vi "DAE Spring Pendulum Simulation_Func.vi"(2 "data":variant, 3 "t":dbl, 4 "X'":dbl[](array[numeric]), 5 "X":dbl[](array[numeric])) -> (0 "error out":errorcluster, 1 "F(X,X',t)":dbl[](array[numeric]))   [LabVIEW 2023]
doc: "DAE Spring Pendulum Simulation Function"
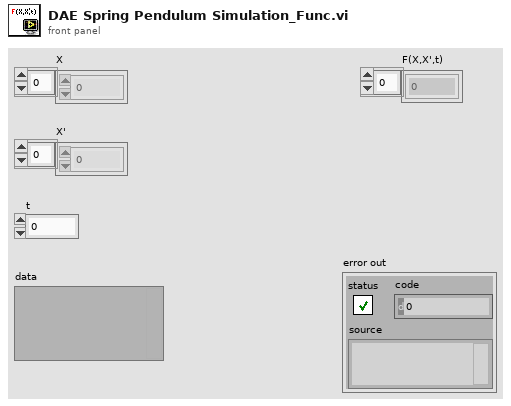
[diagram p1: front panel]
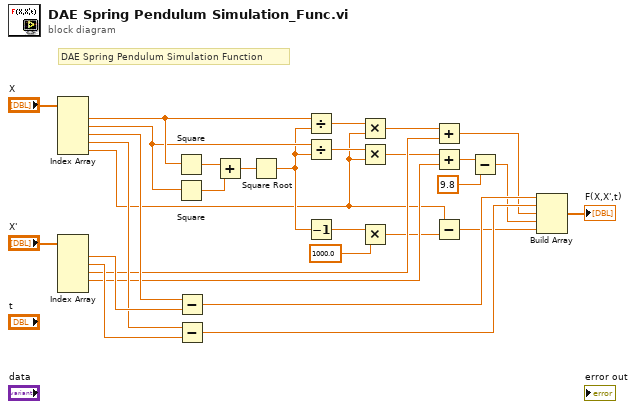
[diagram p0: block diagram]
diagram:
  # "DAE Spring Pendulum Simulation Function"
  n1 = Index Array(array="X") -> (element #1=w24:dbl, element #2=w22:dbl, element #3=w19:dbl, element #4=w18:dbl, element #5=w4:dbl)  [unwired: 5 in]
  n2 = Index Array(array="X'") -> (element #1=w25:dbl, element #2=w23:dbl, element #3=w14:dbl, element #4=w11:dbl)  [unwired: 5 in, 1 out]
  n3 = Square(x=w24) -> (x^2=w28:dbl)
  n4 = Square(x=w22) -> (x^2=w27:dbl)
  n5 = Subtract(x=w19, y=w25) -> (x-y=w21:dbl)
  n6 = Subtract(x=w18, y=w23) -> (x-y=w20:dbl)
  n7 = Add(x=w28, y=w27) -> (x+y=w26:dbl)
  n8 = Square Root(x=w26) -> (sqrt(x)=w7:dbl)
  n9 = Divide(x=w24, y=w7) -> (x/y=w17:dbl)
  n10 = Divide(x=w22, y=w7) -> (x/y=w16:dbl)
  n11 = Decrement(x=w7) -> (x-1=w6:dbl)
  n12 = Multiply(x=w17, y=w4) -> (x*y=w15:dbl)
  n13 = Multiply(x=w16, y=w4) -> (x*y=w12:dbl)
  n14 = Multiply(x=w6, y=1000.0) -> (x*y=w3:dbl)
  n15 = Add(x=w15, y=w14) -> (x+y=w13:dbl)
  n16 = Add(x=w12, y=w11) -> (x+y=w10:dbl)
  n17 = Subtract(x=w4, y=w3) -> (x-y=w2:dbl)
  n18 = Subtract(x=w10, y=9.8) -> (x-y=w8:dbl)
  n19 = Build Array(w21, w20, w13, w8, w2) -> (→"F(X,X',t)":dbl[])
